vi "AddCharacteristic.vi"(8 "error in (no error)":errorcluster, 10 "FullName":string, 11 "Measure in":refnum<class "Measure.lvclass">) -> (0 "error out":errorcluster, 2 "Characteristic":refnum<class "Characteristic.lvclass">, 3 "Measure out":refnum<class "Measure.lvclass">)   [LabVIEW 2021, in "ProligentXMLGenerator.lvlib" / "Measure.lvclass"]
uses:
  Measure.lvclass
  Measure.lvclass/Measure.ctl
  Model/Characteristic/Characteristic.lvclass
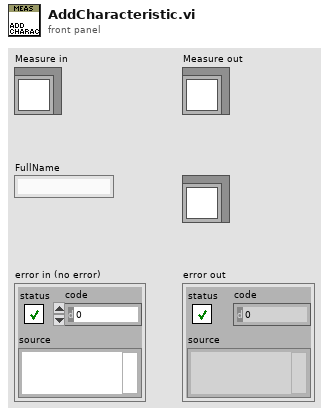
[diagram p1: front panel]
types:
  T1 = typedef "ProligentXMLGenerator.lvlib/Measure.lvclass/Data.ctl" = cluster{"Name":string, "Type":refnum<class "MeasureKind.lvclass">, "Precision":refnum<class "UnsignedByte.lvclass">, "Limit":refnum<class "MeasureLimit.lvclass">, "Characteristics":refnum<class "Characteristic.lvclass">[], "FailureReferences":refnum<class "FailureReference.lvclass">[], "CustomData":refnum<class "CustomData.lvclass">, "MeasureId":refnum<class "Guid.lvclass">, "MeasureTime":refnum<class "DateTime.lvclass">, "Comments":refnum<class "NonNullableString_TruncateAt_255.lvclass">, "Unit":refnum<class "NonEmptyString_30.lvclass">, "Symbol":refnum<class "NonEmptyString_20.lvclass">, "MeasureExecutionStatus":refnum<class "ExecutionStatus.lvclass">}
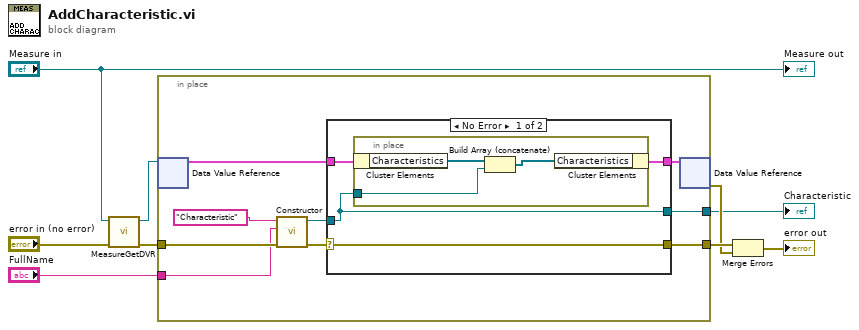
[diagram p0: block diagram]
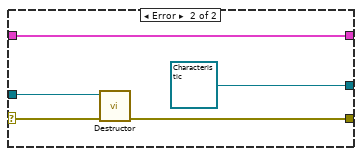
[diagram p2: hidden frame]
diagram:
  n1 = call "MeasureGetDVR.vi"("error in"="error in (no error)", "Measure"="Measure in") -> ("error out"=w8:errorcluster, "DVRReference"=w7:refnum<data-value>)  [unwired: 8 in]
  n2 = in-place "In Place Element Structure" {
    in-place-border: [w18] -> w9
    in-place-border: w8 -> [w11]
    in-place-border: [w15] -> w4
    in-place-border: "FullName" -> [w10]
    n3 = in-place-dvr #1(w7) -> (w17:T1)  [unwired: 1 out]
    n4 = call "Constructor.vi"("error in"=w11, "FullName"=w10, "Name"="Characteristic") -> ("error out"=w13:errorcluster, "Document out"=w14:refnum<class "Characteristic.lvclass">)  [unwired: 7 in]
    n5 = case shown="No Error" w13 {
      selector: w13 -> [w22 w29]
      tunnel: [w19 w30] -> w16
      tunnel: [w22 w28] -> w18
      tunnel: w14 -> [w21 w27]
      tunnel: w17 -> [w20 w30]
      tunnel: [w21 refnum<class "Characteristic.lvclass"> refnum ("ProligentResultProcessor:Characteristic")] -> w15
      frame No Error {
        n6 = in-place "In Place Element Structure" {
          in-place-border: w21 -> [w25]
          n7 = in-place-cluster #2(w20) -> ("Characteristics"=w24:refnum<class "Characteristic.lvclass">[])
          n8 = Build Array (concatenate)(w24, w25) -> (w23:refnum<class "Characteristic.lvclass">[])
          n9 = in-place-cluster #2("Characteristics"=w23) -> (w19:T1)
        }
      }
      frame Error {
        n10 = call "Destructor.vi"("error in"=w29, "Document in"=w27) -> ("error out"=w28:errorcluster)  [unwired: 9 in]
      }
    }
    n11 = in-place-dvr #1(w16) -> (w6:errorcluster)  [unwired: 1 out]
  }
  "Characteristic" <- w4
  n12 = Merge Errors(w9, w6) -> (→"error out":errorcluster)
  "Measure out" <- "Measure in"
